vi "Keysight6700 Main.vi"() -> ()   [LabVIEW 2021]
uses:
  Controls/PS States.ctl
panel:
  in  "Setting":T1={"Max Volt"=10.0, "Voltage Set"=0.01, "Current Lim"=0.5, "Source Type"=enum."Current", "Current Set"=0.01, "Max Current"=10.0, "Voltage Lim"=0.5}
  out "Connect?":bool
  in  "stop":bool
  out "error out":errorcluster
  out "Measurement":dbl=nan
  in  "Enable Output":bool=TRUE
  in  "Alias":string="PS1"
  # "Voltage Src"
  # "Current Src"
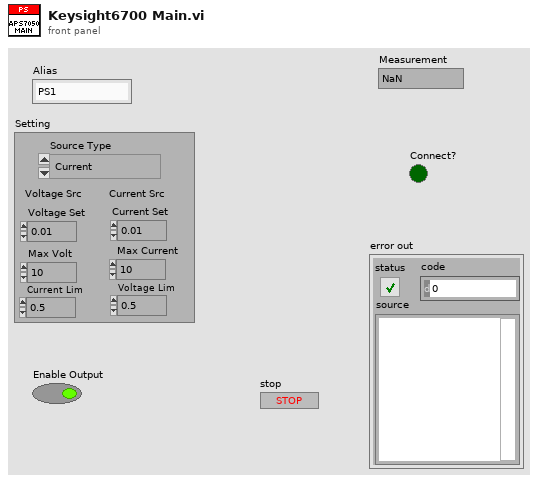
[diagram p1: front panel]
types:
  T1 = cluster{"Max Volt":dbl, "Voltage Set":dbl, "Current Lim":dbl, "Source Type":enum16{"Voltage", "Current"}, "Current Set":dbl, "Max Current":dbl, "Voltage Lim":dbl}
  T2 = typedef "PS States.ctl" = enum16{"Init", "Config", "Enable Output", "Measure", "Close"}
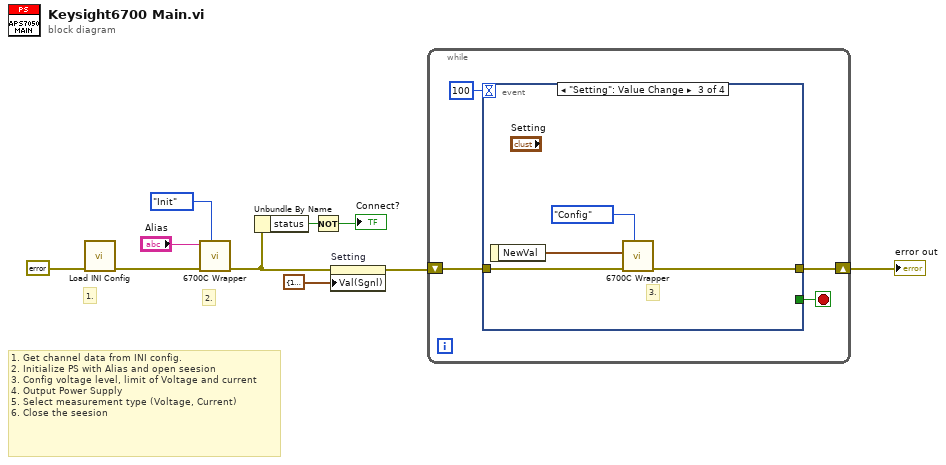
[diagram p0: block diagram]
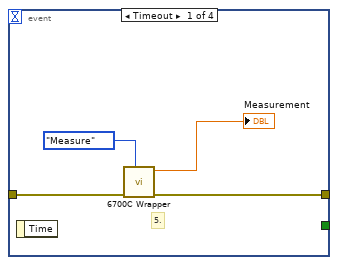
[diagram p2: hidden frame]
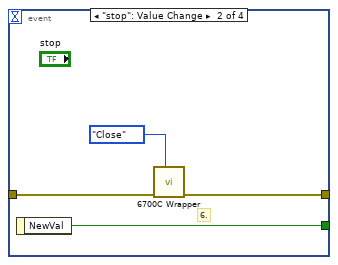
[diagram p3: hidden frame]
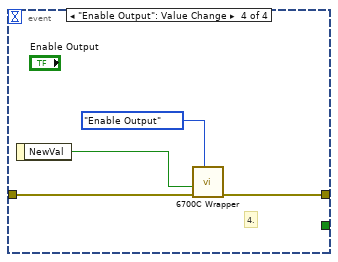
[diagram p4: hidden frame]
diagram:
  # "1. Get channel data from INI config.\n2. Initialize PS with Alias and open seesion \n3. Config voltage level, limit of Voltage and current\n4. Output Power Supply\n5. Select measurement type (Voltage, Current)\n6. Close the seesion"
  # "2."
  # "1."
  n1 = call "Load INI Config.vi"("error in"=errorcluster {"status"=FALSE, "code"=0, "source"=""}) -> ("error out"=w6:errorcluster)  [unwired: 10 in]
  n2 = call "6700C Wrapper.vi"("States"=PS_States."Init", "error in"=w6, "Alias"="Alias") -> ("error out"=w3:errorcluster)  [unwired: 5 in, 3 out]
  n3 = Unbundle By Name(w3) -> ("status"=w5:bool)
  n4 = Not(x=w5) -> (.not. x?=→"Connect?":bool)
  n5 = property on="Setting" class="Clust (strict)"(error in=w3, "Val(Sgnl)"=T1 {"Max Volt"=10.0, "Voltage Set"=5.0, "Current Lim"=0.5, "Source Type"=enum."Voltage", "Current Set"=5.0, "Max Current"=10.0, "Voltage Lim"=0.5} ("Value (Signaling)")) -> (error out=w2:errorcluster)  [unwired: 1 in, 1 out]
  n6 = while {
    shift-right: [w12] -> w9
    shift-left: w2 -> [w13]
    stop <- w14 stop-if-true
    n7 = event shown="[2] \"Setting\": Value Change" {
      selector: _ -> [_ _ _ _]
      dyn-events: _ -> [_ _ _ _]
      timeout: 100 -> [_ _ _ _]
      tunnel: [_ w22 _ _] -> w14
      tunnel: [w16 w20 w25 w29] -> w12
      tunnel: w13 -> [w18 w21 w26 w30]
      event Timeout {
        # "5."
        n8 = event-data() -> ()  [unwired: 1 in, 1 out]
        n9 = call "6700C Wrapper.vi"("States"=PS_States."Measure", "error in"=w18) -> ("error out"=w16:errorcluster, "Measurement"=→"Measurement":dbl)  [unwired: 6 in, 2 out]
      }
      event "stop": Value Change {
        # "6."
        n10 = event-data() -> ("NewVal"=w22:bool)  [unwired: 1 in]
        n11 = call "6700C Wrapper.vi"("States"=PS_States."Close", "error in"=w21) -> ("error out"=w20:errorcluster)  [unwired: 6 in, 3 out]
      }
      event "Setting": Value Change {
        # "3."
        n12 = event-data() -> ("NewVal"=w24:T1)  [unwired: 1 in]
        n13 = call "6700C Wrapper.vi"("States"=PS_States."Config", "error in"=w26, "Setting"=w24) -> ("error out"=w25:errorcluster)  [unwired: 5 in, 3 out]
      }
      event "Enable Output": Value Change {
        # "4."
        n14 = event-data() -> ("NewVal"=w27:bool)  [unwired: 1 in]
        n15 = call "6700C Wrapper.vi"("States"=PS_States."Enable Output", "error in"=w30, "Enable Output"=w27) -> ("error out"=w29:errorcluster)  [unwired: 5 in, 3 out]
      }
    }
  }
  "error out" <- w9
